vi "FTW-Endpoint-Construct.vi"(5 "Endpoint Type":T1, 11 "error in":errorcluster) -> (4 "FTW Endpoint":refnum<class "FTW-Actor-Endpoint.lvclass">, 15 "error out":errorcluster)   [LabVIEW 2013, in "FTW-Actor-Endpoint.lvclass"]
uses:
  FTW-Actor-Endpoint.lvclass
  FTW-Endpoint-Type.ctl
  FTW-Actor-Endpoint.lvclass/FTW-Actor-Endpoint.ctl
panel:
  # "Inputs"
  # "Outputs"
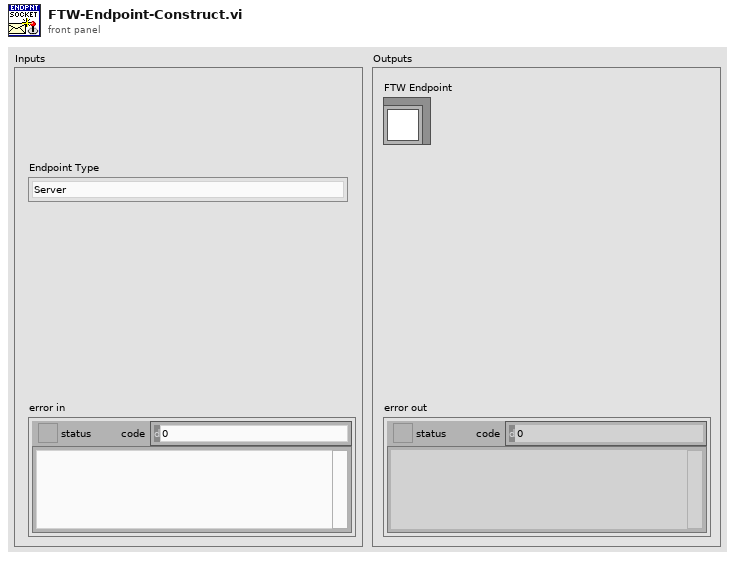
[diagram p1: front panel]
types:
  T1 = typedef "FTW-Actor-Endpoint.lvclass/FTW-Endpoint-Type.ctl" = enum32{"Server", "Client", "Publisher", "Subscriber", "Pipeline Producer", "Pipeline Consumer", "Surveyor", "Respondent", "Exclusive Pair", "Bus"}
  T2 = cluster{"Option":string, "Value":i32, "Comment":string}[]
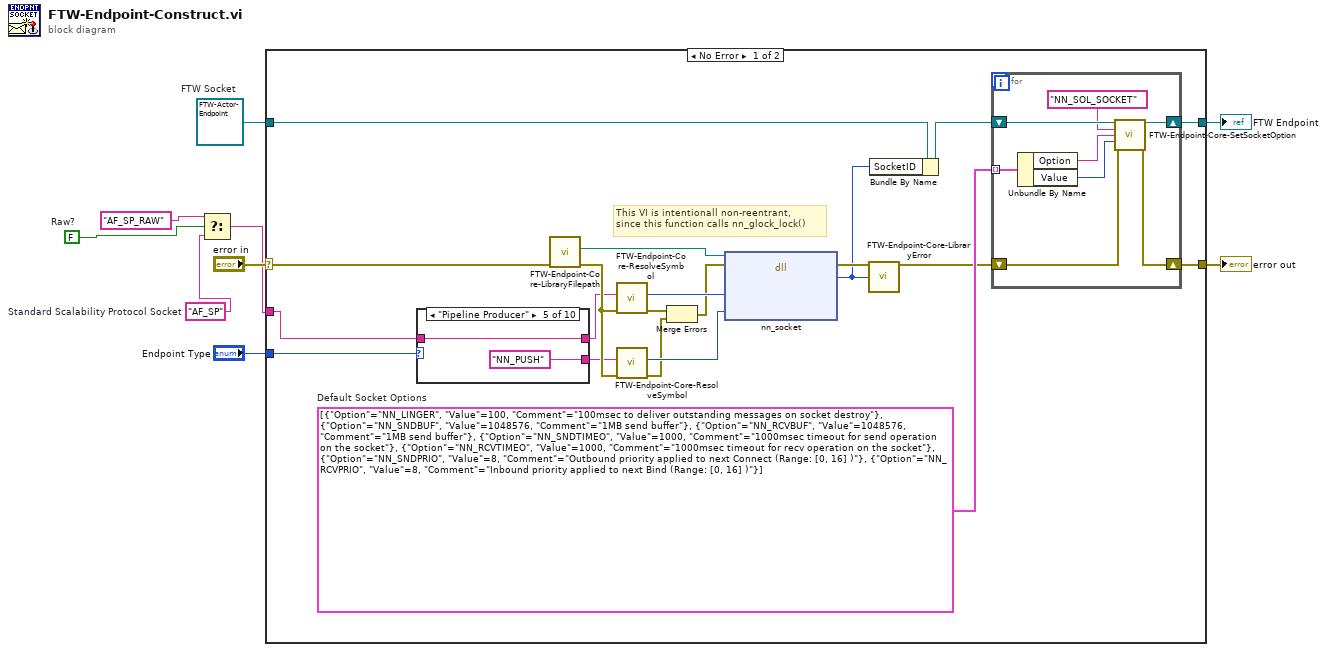
[diagram p0: block diagram]
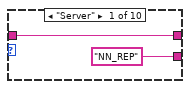
[diagram p2: hidden frame]
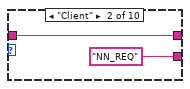
[diagram p3: hidden frame]
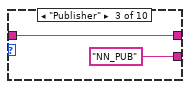
[diagram p4: hidden frame]
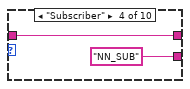
[diagram p5: hidden frame]
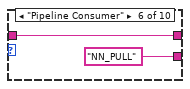
[diagram p6: hidden frame]
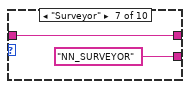
[diagram p7: hidden frame]
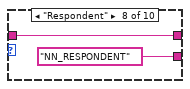
[diagram p8: hidden frame]
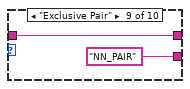
[diagram p9: hidden frame]
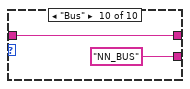
[diagram p10: hidden frame]
diagram:
  w4 = FALSE  # Raw?
  w1 = "AF_SP"  # Standard Scalability Protocol Socket
  w5 = refnum<class "FTW-Actor-Endpoint.lvclass"> refnum  # FTW Socket
  n1 = Select(t="AF_SP_RAW", s=w4, f=w1) -> (s? t:f=w2:string)
  n2 = case shown="No Error" "error in" {
    selector: "error in" -> [w29 w59]
    tunnel: [w16 w58] -> w9
    tunnel: [w17 w59] -> w8
    tunnel: "Endpoint Type" -> [w13 _]
    tunnel: w5 -> [w28 w58]
    tunnel: w2 -> [w10 _]
    frame No Error {
      w18 = T2 [{"Option"="NN_LINGER", "Value"=100, "Comment"="100msec to deliver outstanding messages on socket destroy"}, {"Option"="NN_SNDBUF", "Value"=1048576, "Comment"="1MB send buffer"}, {"Option"="NN_RCVBUF", "Value"=1048576, "Comment"="1MB send buffer"}, {"Option"="NN_SNDTIMEO", "Value"=1000, "Comment"="1000msec timeout for send operation on the socket"}, {"Option"="NN_RCVTIMEO", "Value"=1000, "Comment"="1000msec timeout for recv operation on the socket"}, {"Option"="NN_SNDPRIO", "Value"=8, "Comment"="Outbound priority applied to next Connect (Range: [0, 16] )"}, {"Option"="NN_RCVPRIO", "Value"=8, "Comment"="Inbound priority applied to next Bind (Range: [0, 16] )"}]  # Default Socket Options
      # "This VI is intentionall non-reentrant,\nsince this function calls nn_glock_lock()"
      n3 = case shown="\"Pipeline Producer\"" w13 {
        tunnel: ["NN_REP" "NN_REQ" "NN_PUB" "NN_SUB" "NN_PUSH" "NN_PULL" "NN_SURVEYOR" "NN_RESPONDENT" "NN_PAIR" "NN_BUS"] -> w12
        tunnel: [w30 w32 w34 w36 w38 w40 w42 w44 w46 w48] -> w11
        tunnel: w10 -> [w30 w32 w34 w36 w38 w40 w42 w44 w46 w48]
        frame "Server" {
        }
        frame "Client" {
        }
        frame "Publisher" {
        }
        frame "Subscriber" {
        }
        frame "Pipeline Producer" {
        }
        frame "Pipeline Consumer" {
        }
        frame "Surveyor" {
        }
        frame "Respondent" {
        }
        frame "Exclusive Pair" {
        }
        frame "Bus" {
        }
      }
      n4 = call "FTW-Endpoint-Core-LibraryFilepath.vi"("error in"=w29) -> ("error out"=w24:errorcluster, "Library Filepath"=w27:path)  [unwired: 8 in, 1 out]
      n5 = call "FTW-Endpoint-Core-ResolveSymbol.vi"("error in"=w24, "Symbol"=w11) -> ("error out"=w23:errorcluster, "Symbol Value"=w25:i32)  [unwired: 8 in]
      n6 = call "FTW-Endpoint-Core-ResolveSymbol.vi"("error in"=w24, "Symbol"=w12) -> ("error out"=w22:errorcluster, "Symbol Value"=w26:i32)  [unwired: 8 in]
      n7 = Merge Errors(w23, w22) -> (w21:errorcluster)
      n8 = dll-call lib="?" fn="nn_socket"(path in=w27, error in=w21, "Domain"=w25, "Scalability Protocol"=w26) -> (error out=w20:errorcluster, "Return Value"=w19:i64)  [unwired: 3 in, 1 out]
      n9 = call "FTW-Endpoint-Core-LibraryError.vi"("error in"=w20, "Return Value"=w19) -> ("error out"=w14:errorcluster)  [unwired: 13 in]
      n10 = Bundle By Name(cluster=w28, "SocketID"=w19) -> (w15:refnum<class "FTW-Actor-Endpoint.lvclass">)
      n11 = for {
        tunnel: w18 -> [w57] mode=indexing
        shift-right: [w51] -> w17
        shift-left: w14 -> [w52]
        shift-right: [w56] -> w16
        shift-left: w15 -> [w55]
        n12 = Unbundle By Name(w57) -> ("Option"=w53:string, "Value"=w50:i32)
        n13 = call "FTW-Endpoint-Core-SetSocketOption.vi"("FTW Endpoint"=w55, "Option Level"="NN_SOL_SOCKET", "Option"=w53, "Value"=w50, "error in"=w52) -> ("FTW Endpoint out"=w56:refnum<class "FTW-Actor-Endpoint.lvclass">, "error out"=w51:errorcluster)  [unwired: 9 in]
      }
    }
    frame Error {
    }
  }
  "error out" <- w8
  "FTW Endpoint" <- w9
